vi "load indices.vi"(8 "error in (no error)":errorcluster, 11 "manager_daemon in":refnum<class "manager_daemon.lvclass">) -> (0 "error out":errorcluster, 3 "manager_daemon out":refnum<class "manager_daemon.lvclass">)   [LabVIEW 2024, in "manager_daemon.lvclass"]
uses:
  manager_daemon.lvclass
  type_defs/msg--cluster.ctl
  type_defs/cmd--enum.ctl
  manager_daemon.lvclass/manager_daemon.ctl
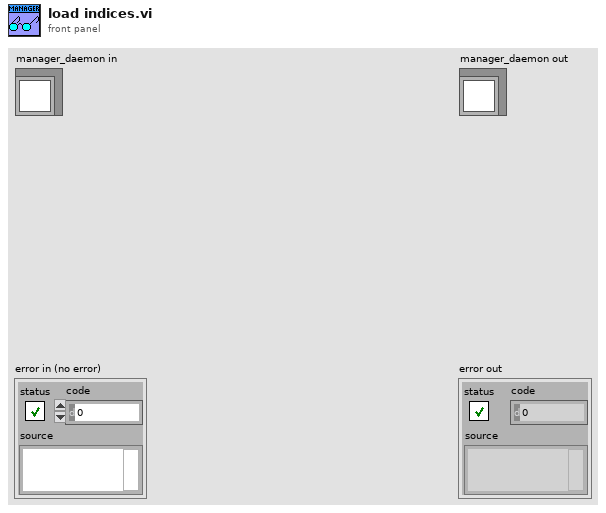
[diagram p1: front panel]
types:
  T1 = typedef "manager_daemon.lvclass/msg--cluster.ctl" = cluster{"cmd":T2, "data":variant}
  T2 = typedef "manager_daemon.lvclass/cmd--enum.ctl" = enum16{"init", "run", "load binaries", "build binaries", "save binaries", "display info", "apply filter", "add volume", "add issues", "add issue", "delete volume", "delete issues", "exit"}
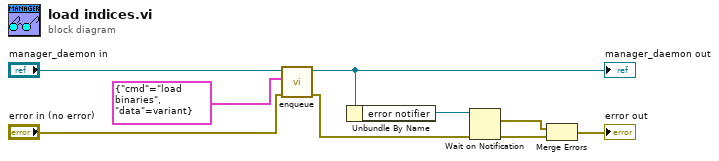
[diagram p0: block diagram]
diagram:
  n1 = call "enqueue.vi"("error in (no error)"="error in (no error)", "msg"=T1 {"cmd"=enum."load binaries", "data"=variant}, "manager_daemon in"="manager_daemon in") -> ("error out"=w4:errorcluster, "manager_daemon out"=w6:refnum<class "manager_daemon.lvclass">)  [unwired: 7 in]
  "manager_daemon out" <- w6
  n2 = Unbundle By Name(w6) -> ("error notifier"=w5:refnum<notifier>)
  n3 = Wait on Notification(notifier=w5, error in (no error)=w4) -> (notification=w3:errorcluster, error out=w2:errorcluster)  [unwired: 2 in, 2 out]
  n4 = Merge Errors(w3, w2) -> (→"error out":errorcluster)
